vi "Slope.vi"(8 "Y2":dbl, 9 "X2":dbl, 10 "Y1":dbl, 11 "X1":dbl) -> (0 "?":string, 1 "Angle (Degrees)":dbl, 2 "Angle (Radians)":dbl, 3 "Linear Slope":dbl)   [LabVIEW 2020]
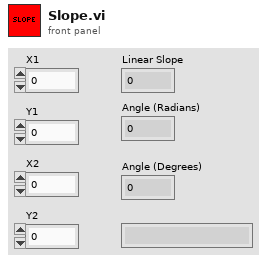
[diagram p1: front panel]
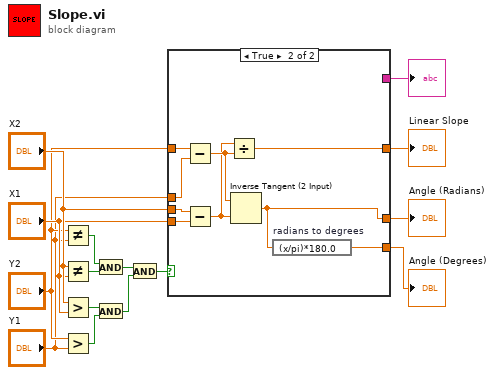
[diagram p0: block diagram]
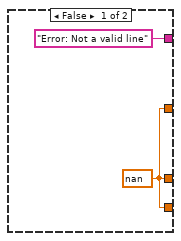
[diagram p2: hidden frame]
diagram:
  n1 = Not Equal?(x="Y2", y="Y1") -> (x != y?=w14:bool)
  n2 = Not Equal?(x="X2", y="X1") -> (x != y?=w13:bool)
  n3 = Greater?(x="X2", y="X1") -> (0:w9:bool)
  n4 = Greater?(x="Y2", y="Y1") -> (0:w5:bool)
  n5 = And(x=w14, y=w13) -> (x .and. y?=w8:bool)
  n6 = And(x=w9, y=w5) -> (x .and. y?=w7:bool)
  n7 = And(x=w8, y=w7) -> (x .and. y?=w6:bool)
  n8 = case shown="True" w6 {
    tunnel: "Y1" -> [_ w26]
    tunnel: "Y2" -> [_ w25]
    tunnel: "X1" -> [_ w24]
    tunnel: "X2" -> [_ w23]
    tunnel: [w16 w22] -> w15
    tunnel: ["Error: Not a valid line" _] -> w12
    tunnel: [w16 w19] -> w11
    tunnel: [w16 w18] -> w10
    frame False {
      w16 = nan
    }
    frame True {
      n9 = Subtract(x=w25, y=w26) -> (x-y=w21:dbl)
      n10 = Subtract(x=w23, y=w24) -> (x-y=w20:dbl)
      n11 = Divide(x=w20, y=w21) -> (x/y=w22:dbl)
      n12 = Inverse Tangent (2 Input)(1:w20, 2:w21) -> (0:w19:dbl)
      n13 = expression code="(x/pi)*180.0" "radians to degrees"(w19) -> (w18:dbl)
    }
  }
  "Linear Slope" <- w15
  "?" <- w12
  "Angle (Radians)" <- w11
  "Angle (Degrees)" <- w10
